vi "Drive Global.vi"() -> ()   [LabVIEW 2019]
uses:
  Drive Mode Typedef.ctl
  Drive Command Typedef.ctl
  Calculations or utilities/Is command done typedef.ctl
panel:
  out "Drive Command Done?":T1
  out "Drive Right Sensors":T2
  out "Drive Left Sensors":T3
  in  "Drive Auton Command":T4
  in  "Drive Teleop Command":T4
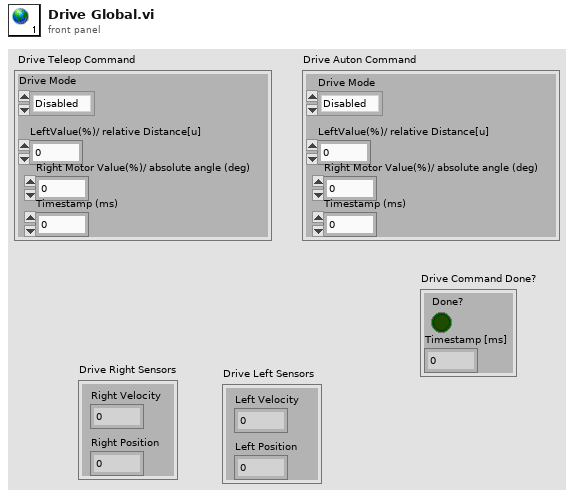
[diagram p1: front panel]
types:
  T1 = typedef "Is command done typedef.ctl" = cluster{"Done?":bool, "Timestamp [ms]":dbl}
  T2 = cluster{"Right Velocity":dbl, "Right Position":dbl}
  T3 = cluster{"Left Velocity":dbl, "Left Position":dbl}
  T4 = typedef "Drive Command Typedef.ctl" = cluster{"Drive Mode":T5, "LeftValue(%)/ relative Distance[u]":dbl, "Right Motor Value(%)/ absolute angle (deg)":dbl, "Timestamp (ms)":dbl}
  T5 = typedef "Drive Mode Typedef.ctl" = enum16{"Disabled", "Auto-align", "Drive Distance", "Turn to angle", "Driver"}
diagram:
